vi "Vision Processing.vi"(4 "error in (no error)":errorcluster, 7 "Image Size":T1=enum."320x240") -> ()   [LabVIEW 2015]
uses:
  Vision Support Code/Camera Types.ctl
  <vilib>/Rock Robotics/WPI/Camera/WPI_CameraImageSize.ctl
  <vilib>/Rock Robotics/WPI/Camera/WPI_CameraWhite Balance Values.ctl
  <vilib>/Rock Robotics/WPI/Camera/WPI_CameraExposure Values.ctl
  <vilib>/Rock Robotics/WPI/Camera/WPI_CameraFrameRate.ctl
  Robot Global Data.vi
  <vilib>/vision/NI_Vision_Development_Module.lvlib
panel:
  in  "Image Size 2":T1=enum."320x240"
  out "Highest Avg Score":dbl
  in  "Min Score Threshold":i32=75
  out "Detected Targets":T2(array[cluster]) {"Normalized Rect"."Numeric 5" format="%#_2g"; "Normalized Rect"."Numeric 3" format="%#_2g"; "Normalized Rect"."Numeric 2" format="%#_2g"; "Normalized Rect"."Numeric" format="%#_2g"}
  out "Sorted Particle Scores":T3(array[cluster]) {"Moment Factor" format="%#_3g"; "Aspect Ratio" format="%#_3g"; "Area to CH" format="%#_3g"; "X" format="%#_3g"; "Y" format="%#_3g"}
  in  "Display Original":bool=TRUE
  in  "Display Mask":bool=TRUE
  out "fps":dbl
  in  "Emphasize Limit Tests":bool=TRUE
  in  "Camera Type":T4=enum."MS HD3000 square"
  in  "Aspect Fudge Factor":dbl=1.0
  in  "Score Threshold":dbl=75.0
  out "ms to process":u32
  out "Qualified Particles":i32
  in  "LED Color":T5={"Hue"={23.67058792990901, 48.923317529462665}, "Sat"={66.78571428571429, 255.0}, "Val"={48.571428571428584, 255.0}} {"Hue" scale=0.0..255.0 scale format="%#_3g"}
  out "Masked":T6(plugin-control)
  out "Original Image":T6(plugin-control)
  # "This is only the initial camera size.\nOther camera setup is done\non the diagram. Notice it is set\nonce before the loop but can be\nupdated within the loop if needed."
  # "Instructions:\nUse LED Color to threshold and build particles. Adjust calibration if needed.\nDisplays are very useful for debugging, but will slow down execution, so you\nmay want to disable once working.\nAnnotations show the rectangle and the scores from top to bottom.\nChange camera setting on diagram."
  # "Density Profile"
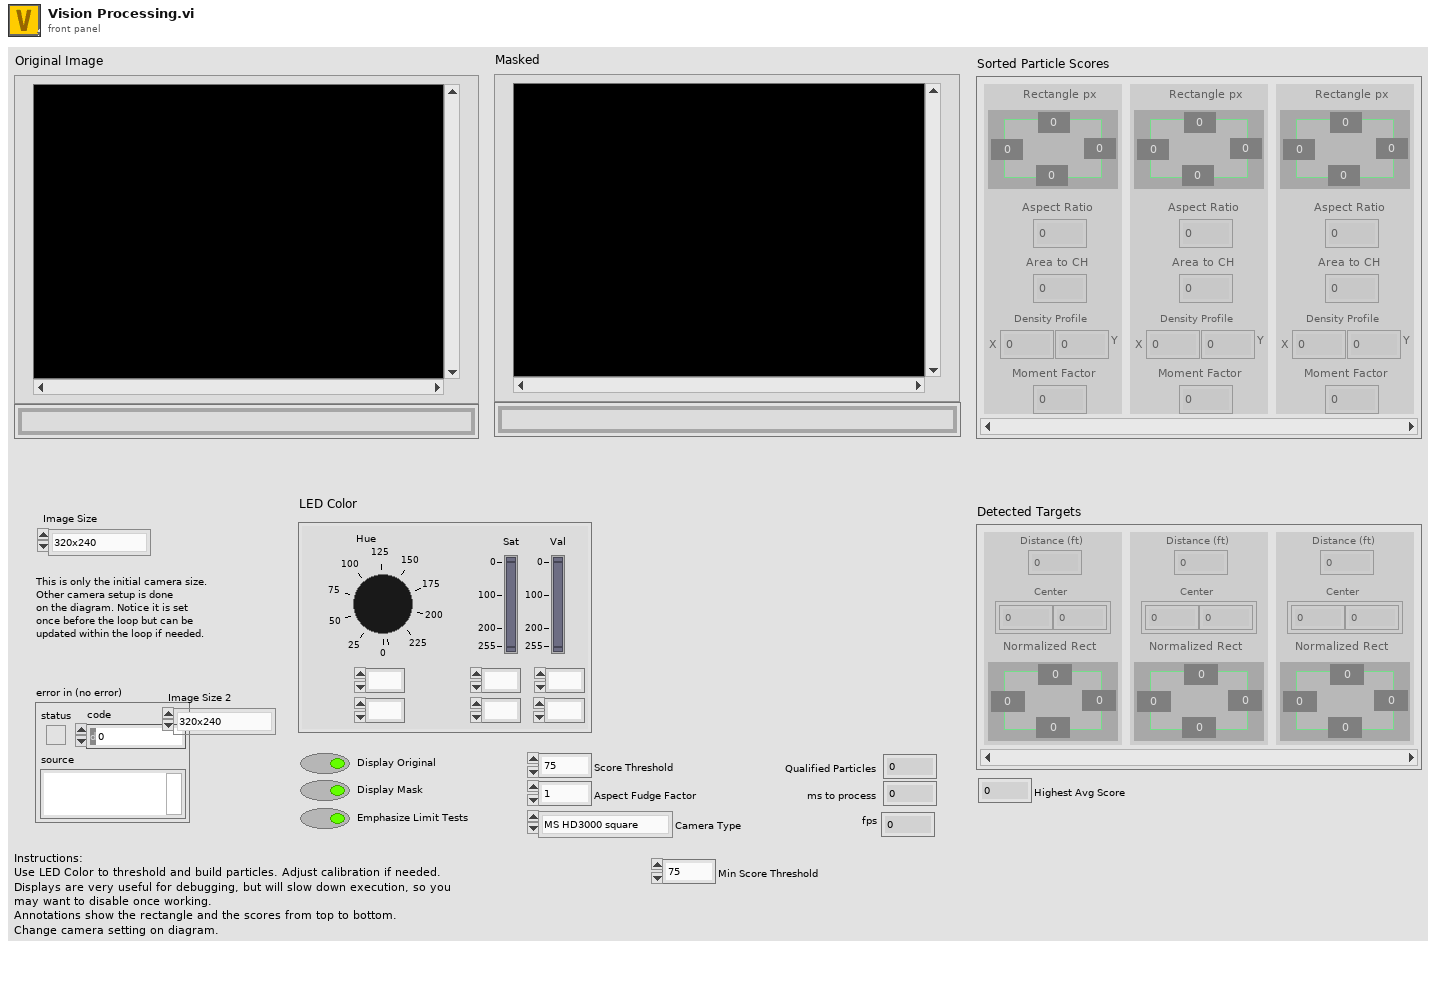
[diagram p1: front panel]
types:
  T1 = typedef "WPI_CameraImageSize.ctl" = enum16{"640x480", "320x240", "160x120", "Custom"}
  T2 = cluster{"Distance (ft)":dbl, "Center":cluster{dbl, dbl}, "Normalized Rect":cluster{"Numeric":dbl, "Numeric 2":dbl, "Numeric 3":dbl, "Numeric 5":dbl}}[]
  T3 = cluster{"Rectangle px":cluster{"Numeric":dbl, "Numeric 2":dbl, "Numeric 3":dbl, "Numeric 5":dbl}, "Aspect Ratio":dbl, "Area to CH":dbl, "X":dbl, "Y":dbl, "Moment Factor":dbl}[]
  T4 = typedef "Camera Types.ctl" = enum16{"206", "1011", "1013", "MS HD3000 square", "MS HD3000 640x480"}
  T5 = cluster{"Hue":cluster{dbl, dbl}, "Sat":cluster{dbl, dbl}, "Val":cluster{dbl, dbl}}
  T6 = typedef "IMAQ Image.ctl" = refnum<image>
  T7 = typedef "WPI_CameraFrameRate.ctl" = u32
  T8 = typedef "WPI_CameraExposure Values.ctl" = enum16{"Auto", "Flicker-free 50 Hz", "Flicker-free 60 Hz", "Hold current", "Custom"}
  T9 = typedef "WPI_CameraWhite Balance Values.ctl" = enum16{"Auto", "Fixed indoor", "Fixed outdoor 1", "Fixed outdoor 2", "Fixed fluorescent 1", "Fixed fluorescent 2", "Hold current", "Custom"}
  T10 = typedef "Particle Parameters" = i32
  T11 = typedef "Image Type" = u32
  T12 = typedef "WPI_CameraDevRef.ctl" = cluster{"Camera Address":string, "CameraStatus":errorcluster}
  T13 = cluster{"Bounding box":cluster{"left":dbl, "top":dbl, "right":dbl, "bottom":dbl}, "Aspect Ratio":dbl, "Area to CH":dbl, "X Mask":dbl, "Y Mask":dbl, "Moment":dbl}[]
  T14 = cluster{"Rectangle":cluster{"Numeric":dbl, "Numeric 2":dbl, "Numeric 3":dbl, "Numeric 5":dbl}, "L":dbl, "Area to CH":dbl, "X":dbl, "Y":dbl, "Moment Factor":dbl}[]
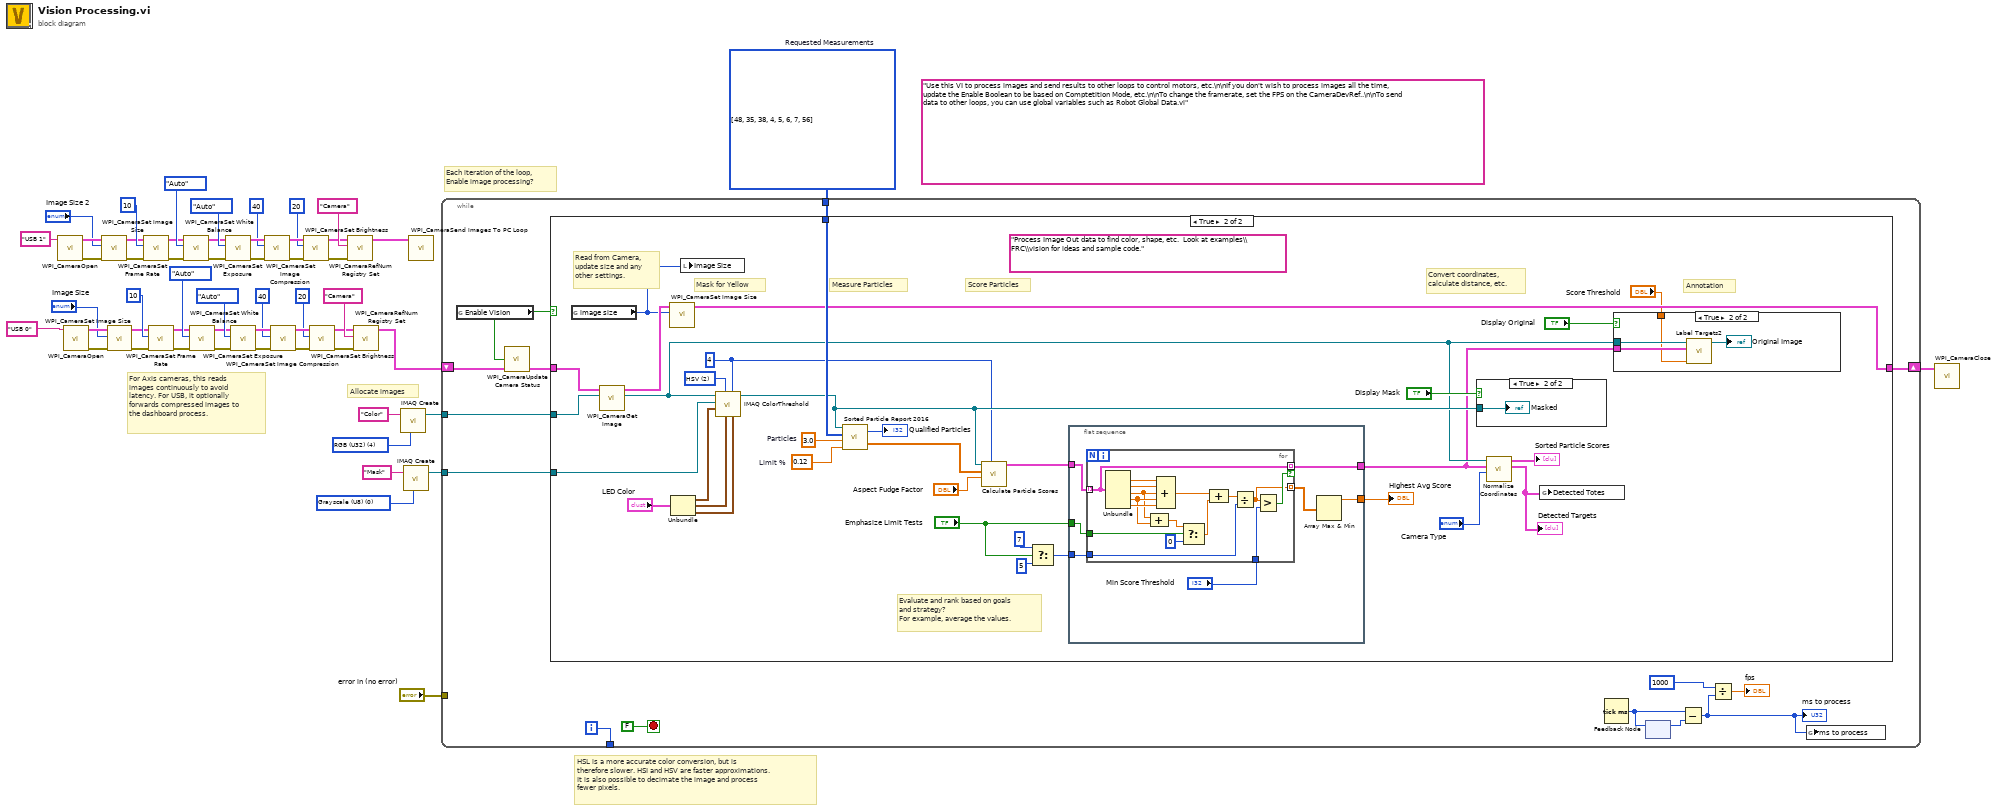
[diagram p0: block diagram]
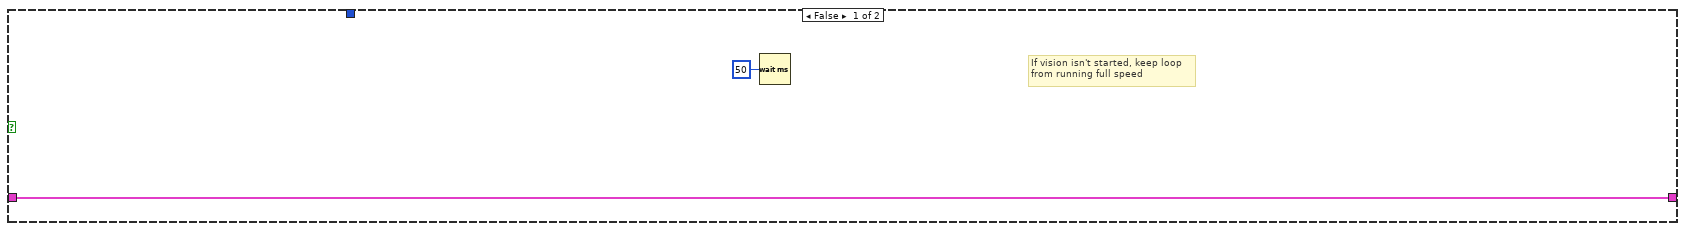
[diagram p2: hidden frame]
diagram:
  (unwired) "Use this VI to process images and send results to other loops to control motors, etc.\n\nIf you don't wish to process images all the time, update the Enable Boolean to be based on Comptetition Mode, etc.\n\nTo change the framerate, set the FPS on the CameraDevRef..\n\nTo send data to other loops, you can use global variables such as Robot Global Data.vi"
  w49 = T10[] [48, 35, 38, 4, 5, 6, 7, 56] items=["Center of Mass X", "Center of Mass Y", "First Pixel X", "First Pixel Y", "Bounding Rect Left", "Bounding Rect Top", "Bounding Rect Right", "Bounding Rect Bottom", "Max Feret Diameter Start X", "Max Feret Diameter Start Y", "Max Feret Diameter End X", "Max Feret Diameter End Y", "Max Horiz. Segment Length Left", "Max Horiz. Segment Length Right", "Max Horiz. Segment Length Row", "-", "Bounding Rect Width", "Bounding Rect Height", "Bounding Rect Diagonal", "Perimeter", "Convex Hull Perimeter", "Holes' Perimeter", "Max Feret Diameter", "Equivalent Ellipse Major Axis", "Equivalent Ellipse Minor Axis", "Equivalent Ellipse Minor Axis (Feret)", "Equivalent Rect Long Side", "Equivalent Rect Short Side", "Equivalent Rect Diagonal", "Equivalent Rect Short Side (Feret)", "Average Horiz. Segment Length", "Average Vert. Segment Length", "Hydraulic Radius", "Waddel Disk Diameter", "-", "Area", "Holes' Area", "Particle & Holes' Area", "Convex Hull Area", "Image Area", "-", "Number of Holes", "Number of Horiz. Segments", "Number of Vert. Segments", "-", "Orientation", "Max Feret Diameter Orientation", "-", "% Area/Image Area", "% Area/(Particle & Holes' Area)", "Ratio of Equivalent Ellipse Axes", "Ratio of Equivalent Rect Sides", "-", "Elongation Factor", "Compactness Factor", "Heywood Circularity Factor", "Type Factor", "-", "Sum X", "Sum Y", "Sum XX", "Sum XY", "Sum YY", "Sum XXX", "Sum XXY", "Sum XYY", "Sum YYY", "-", "Moment of Inertia XX", "Moment of Inertia XY", "Moment of Inertia YY", "Moment of Inertia XXX", "Moment of Inertia XXY", "Moment of Inertia XYY", "Moment of Inertia YYY", "Norm. Moment of Inertia XX", "Norm. Moment of Inertia XY", "Norm. Moment of Inertia YY", "Norm. Moment of Inertia XXX", "Norm. Moment of Inertia XXY", "Norm. Moment of Inertia XYY", "Norm. Moment of Inertia YYY", "Hu Moment 1", "Hu Moment 2", "Hu Moment 3", "Hu Moment 4", "Hu Moment 5", "Hu Moment 6", "Hu Moment 7"]  # Requested Measurements
  w52 = T11 0 items=["Grayscale (U8)", "Grayscale (I16)", "Grayscale (SGL)", "Complex (CSG)", "RGB (U32)", "HSL (U32)", "RGB (U64)", "Grayscale (U16)"] ("Image Type")
  w54 = T11 4 items=["Grayscale (U8)", "Grayscale (I16)", "Grayscale (SGL)", "Complex (CSG)", "RGB (U32)", "HSL (U32)", "RGB (U64)", "Grayscale (U16)"] ("Image Type")
  # "Each iteration of the loop,\nEnable image processing?"
  # "HSL is a more accurate color conversion, but is\ntherefore slower. HSI and HSV are faster approximations.\nIt is also possible to decimate the image and process\nfewer pixels."
  # "For Axis cameras, this reads\nimages continuously to avoid\nlatency. For USB, it optionally\nforwards compressed images to\nthe dashboard process."
  # "Allocate images"
  n1 = call <vilib>:"WPI_CameraOpen.vi"("Camera Address"="USB 1") -> ("error out"=w15:errorcluster, "CameraDevRef"=w14:T12)  [unwired: 1 in, 8 out]
  n2 = call <vilib>:"WPI_CameraOpen.vi"("Camera Address"="USB 0" ("format string")) -> ("error out"=w39:errorcluster, "CameraDevRef"=w38:T12)  [unwired: 1 in, 8 out]
  n3 = call <vilib>:"WPI_CameraSet Image Size.vi"("error in (no error)"=w15, "Image Size"="Image Size 2", "CameraDevRef"=w14) -> ("error out"=w16:errorcluster, "CameraDevRef Out"=w13:T12)  [unwired: 1 in, 6 out]
  n4 = call <vilib>:"WPI_CameraSet Image Size.vi"("error in (no error)"=w39, "Image Size"="Image Size", "CameraDevRef"=w38) -> ("error out"=w40:errorcluster, "CameraDevRef Out"=w37:T12)  [unwired: 1 in, 6 out]
  n5 = call <vilib>:"WPI_CameraSet Frame Rate.vi"("error in (no error)"=w16, "Frame Rate (fps)"=T7 10, "CameraDevRef"=w13) -> ("error out"=w17:errorcluster, "CameraDevRef Out"=w11:T12)  [unwired: 7 out]
  n6 = call <vilib>:"WPI_CameraSet Frame Rate.vi"("error in (no error)"=w40, "Frame Rate (fps)"=T7 10, "CameraDevRef"=w37) -> ("error out"=w41:errorcluster, "CameraDevRef Out"=w35:T12)  [unwired: 7 out]
  n7 = call <vilib>:"WPI_CameraSet White Balance.vi"("error in (no error)"=w17, "White Balance"=WPI_CameraWhite_Balance_Values."Auto", "CameraDevRef"=w11) -> ("error out"=w18:errorcluster, "CameraDevRef Out"=w12:T12)  [unwired: 1 in, 6 out]
  n8 = call <vilib>:"WPI_CameraSet White Balance.vi"("error in (no error)"=w41, "White Balance"=WPI_CameraWhite_Balance_Values."Auto", "CameraDevRef"=w35) -> ("error out"=w42:errorcluster, "CameraDevRef Out"=w36:T12)  [unwired: 1 in, 6 out]
  n9 = call <vilib>:"WPI_CameraSet Exposure.vi"("error in (no error)"=w18, "Exposure"=WPI_CameraExposure_Values."Auto", "CameraDevRef"=w12) -> ("error out"=w19:errorcluster, "CameraDevRef Out"=w9:T12)  [unwired: 1 in, 6 out]
  n10 = call <vilib>:"WPI_CameraSet Exposure.vi"("error in (no error)"=w42, "Exposure"=WPI_CameraExposure_Values."Auto", "CameraDevRef"=w36) -> ("error out"=w43:errorcluster, "CameraDevRef Out"=w33:T12)  [unwired: 1 in, 6 out]
  n11 = call <vilib>:"WPI_CameraSet Image Compression.vi"("error in (no error)"=w19, "Compression"=40, "CameraDevRef"=w9) -> ("error out"=w20:errorcluster, "CameraDevRef Out"=w10:T12)  [unwired: 7 out]
  n12 = call <vilib>:"WPI_CameraSet Image Compression.vi"("error in (no error)"=w43, "Compression"=40, "CameraDevRef"=w33) -> ("error out"=w44:errorcluster, "CameraDevRef Out"=w34:T12)  [unwired: 7 out]
  n13 = call <vilib>:"WPI_CameraSet Brightness.vi"("error in (no error)"=w20, "Brightness"=20, "CameraDevRef"=w10) -> ("error out"=w21:errorcluster, "CameraDevRef Out"=w4:T12)  [unwired: 7 out]
  n14 = call <vilib>:"WPI_CameraSet Brightness.vi"("error in (no error)"=w44, "Brightness"=20, "CameraDevRef"=w34) -> ("error out"=w45:errorcluster, "CameraDevRef Out"=w26:T12)  [unwired: 7 out]
  n15 = call <vilib>:"WPI_CameraRefNum Registry Set.vi"("error in (no error)"=w21, "refnum name"="Camera", "CameraDevRef"=w4) -> ("CameraDevRef"=w2:T12)  [unwired: 1 in, 7 out]
  n16 = call <vilib>:"WPI_CameraRefNum Registry Set.vi"("error in (no error)"=w45, "refnum name"="Camera", "CameraDevRef"=w26) -> ("CameraDevRef"=w25:T12)  [unwired: 1 in, 7 out]
  n17 = call "IMAQ Create"("Image Name"="Color", "Image Type"=w54) -> ("New Image"=w53:T6)  [unwired: 2 in, 2 out]
  n18 = call "IMAQ Create"("Image Name"="Mask", "Image Type"=w52) -> ("New Image"=w50:T6)  [unwired: 2 in, 2 out]
  n19 = call <vilib>:"WPI_CameraSend Images To PC Loop.vi"("CameraDevRef"=w2) -> ()  [unwired: 11 in]
  n20 = while {
    tunnel: w53 -> [w64]
    tunnel: w50 -> [w68]
    tunnel: w49 -> [w67]
    tunnel: "error in (no error)" -> [_]
    tunnel: [w63] -> _
    shift-right: [w59] -> w27
    shift-left: w25 -> [w61]
    i -> [w63]
    stop <- FALSE stop-if-true
    n21 = global read "Robot Global Data.vi" "Enable Vision"() -> (w62:bool)
    n22 = call <vilib>:"WPI_CameraUpdate Camera Status.vi"("CameraDevRef In"=w61, "Enable Vision"=w62) -> ("CameraDevRef Out"=w60:T12)  [unwired: 3 in]
    n23 = case shown="True" w62 {
      tunnel: w68 -> [_ w104]
      tunnel: w67 -> [_ w99]
      tunnel: w60 -> [w70 w95]
      tunnel: w64 -> [_ w94]
      tunnel: [w70 w92] -> w59
      frame False {
        # "If vision isn't started, keep loop\nfrom running full speed"
        n24 = Wait (ms)(milliseconds to wait=u32 50) -> ()  [unwired: 1 out]
      }
      frame True {
        w75 = 4 ("Replace Value")
        w89 = u16 2 items=["RGB", "HSL", "HSV", "HSI"] ("Color Mode")
        (unwired) "Process Image Out data to find color, shape, etc.  Look at examples\\FRC\\vision for ideas and sample code."
        w96 = 0.12  # Limit %
        w98 = 3.0  # Particles
        # "Evaluate and rank based on goals\nand strategy?\nFor example, average the values."
        # "Read from Camera,\nupdate size and any\nother settings."
        # "Measure Particles"
        # "Convert coordinates,\ncalculate distance, etc."
        # "Annotation"
        # "Score Particles"
        # "Mask for Yellow"
        n25 = global read "Robot Global Data.vi" "image size"() -> (w73:T1)
        n26 = call <vilib>:"WPI_CameraGet Image.vi"("Image"=w94, "CameraDevRef"=w95) -> ("Image Out"=w78:T6, "CameraDevRef Out"=w93:T12)  [unwired: 7 in, 1 out]
        n27 = call <vilib>:"WPI_CameraSet Image Size.vi"("Image Size"=w73, "CameraDevRef"=w93) -> ("CameraDevRef Out"=w92:T12)  [unwired: 2 in, 7 out]
        n28 = Unbundle("LED Color") -> ("Hue"=w103:cluster{dbl, dbl}, "Sat"=w102:cluster{dbl, dbl}, "Val"=w101:cluster{dbl, dbl})
        n29 = local write "Image Size"(w73) -> ()
        n30 = call "IMAQ ColorThreshold"("Blue or Luma or Val or Inten Range"=w101, "Replace Value"=w75, "Green or Sat Range"=w102, "Color Mode"=w89, "Red or Hue Range"=w103, "Image Dst"=w104, "Image Src"=w78) -> ("Image Dst Out"=w88:T6)  [unwired: 3 in, 1 out]
        n31 = call "Sorted Particle Report 2016.vi"("Min Area Size %"=w96, "Particle Count Limit"=w98, "Pixel Measurements"=w99, "Image in"=w88) -> ("Sorted Data"=w87:dbl[][], "Particles"=→"Qualified Particles":i32)
        n32 = call "Calculate Particle Scores.vi"("Pixel Value"=w75, "Aspect Fudge Factor"="Aspect Fudge Factor", "Sorted Data"=w87, "Image in"=w88) -> ("Scores"=w85:T13)  [unwired: 7 in]
        n33 = Select(t=7, s="Emphasize Limit Tests", f=5) -> (s? t:f=w82:i32)
        n34 = flat-sequence {
          tunnel: w85 -> [w115]
          tunnel: w82 -> [w113]
          tunnel: [w116] -> w81
          tunnel: [w110] -> w77
          tunnel: "Emphasize Limit Tests" -> [w114]
          frame #0 {
            n35 = for {
              tunnel: w115 -> [w130] mode=indexing
              tunnel: [w130] -> w110 mode=indexing if=w129
              tunnel: [w128] -> w111 mode=indexing
              tunnel: w113 -> [w127]
              tunnel: "Min Score Threshold" -> [w126]
              tunnel: w114 -> [w119]
              n36 = Unbundle(w130) -> ("Aspect Ratio"=w132:dbl, "Area to CH"=w131:dbl, "X Mask"=w121:dbl, "Y Mask"=w122:dbl, "Moment"=w123:dbl)  [unwired: 1 out]
              n37 = Compound Arithmetic op=ADD(w121, w122) -> (w120:dbl)
              n38 = Compound Arithmetic op=ADD(w132, w131, w121, w122, w123) -> (w125:dbl)
              n39 = Select(t=w120, s=w119, f=0) -> (s? t:f=w118:dbl)
              n40 = Compound Arithmetic op=ADD(w125, w118) -> (w124:dbl)
              n41 = Divide(x=w124, y=w127) -> (x/y=w128:dbl)
              n42 = Greater?(x=w128, y=w126) -> (0:w129:bool)
            }
            n43 = Array Max & Min(array=w111) -> (max value=w116:dbl)  [unwired: 3 out]
          }
        }
        n44 = case shown="True" "Display Mask" {
          tunnel: w88 -> [_ w109]
          frame False {
          }
          frame True {
            "Masked" <- w109
          }
        }
        n45 = call "Normalize Coordinates.vi"("Camera Type"="Camera Type", "Targets"=w77, "Image in"=w78) -> ("Found Targets"=w74:T2, "Sorted Scores"=→"Sorted Particle Scores":T14)  [unwired: 7 in]
        "Detected Targets" <- w74
        n46 = global write "Robot Global Data.vi" "Detected Totes"(w74) -> ()
        n47 = case shown="True" "Display Original" {
          tunnel: w78 -> [_ w108]
          tunnel: w77 -> [_ w106]
          tunnel: "Score Threshold" -> [_ w105]
          frame False {
          }
          frame True {
            n48 = call "Label Targets2.vi"("Score Threshold"=w105, "Targets"=w106, "Image in"=w108) -> ("Image out"=→"Original Image":T6)  [unwired: 8 in]
          }
        }
        "Highest Avg Score" <- w81
      }
    }
    n49 = Tick Count (ms)() -> (millisecond timer value=w65:u32)
    n50 = feedback-in #1(w65) -> ()
    n51 = feedback #1() -> (w66:u32)  [unwired: 1 in]
    n52 = Subtract(x=w65, y=w66) -> (x-y=w58:u32)
    "ms to process" <- w58
    n53 = Divide(x=1000 ("Brightness"), y=w58) -> (x/y=→"fps":dbl)
    n54 = global write "Robot Global Data.vi" "ms to process"(w58) -> ()
  }
  n55 = call <vilib>:"WPI_CameraClose.vi"("CameraDevRef"=w27) -> ()  [unwired: 1 in, 10 out]
